vi "Write Path.vi"(8 "error in (no error)":errorcluster, 10 "Path":path, 11 "ElectrometerError in":refnum<class "ElectrometerError.lvclass">) -> (0 "error out":errorcluster, 3 "ElectrometerError out":refnum<class "ElectrometerError.lvclass">)   [LabVIEW 2016, in "ElectrometerError.lvclass"]
uses:
  ElectrometerError.lvclass
  ElectrometerError.lvclass/ElectrometerError.ctl
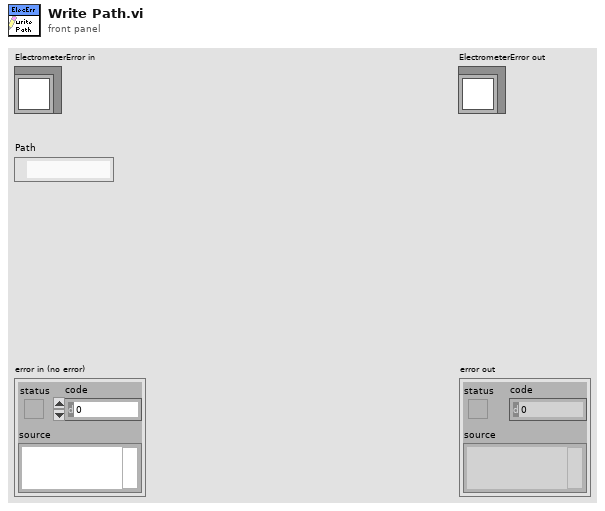
[diagram p1: front panel]
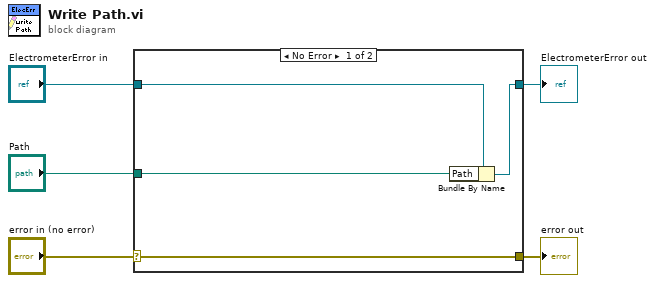
[diagram p0: block diagram]
diagram:
  n1 = case shown="No Error" "error in (no error)" {
    selector: "error in (no error)" -> [w9 w10]
    tunnel: [w9 w10] -> w4
    tunnel: [w7 w11] -> w2
    tunnel: "ElectrometerError in" -> [w8 w11]
    tunnel: "Path" -> [w6 _]
    frame No Error {
      n2 = Bundle By Name(cluster=w8, "Path"=w6) -> (w7:refnum<class "ElectrometerError.lvclass">)
    }
    frame Error {
    }
  }
  "error out" <- w4
  "ElectrometerError out" <- w2
